vi "Initialize Daemon.vi"(8 "error in":errorcluster, 9 "Data Model":refnum<class "Device Data Model.lvclass">, 10 "transmission data unit":refnum<class "Transmission Data Unit.lvclass">, 11 "TCP slave in":refnum<class "TCP Slave.lvclass">) -> (0 "error out":errorcluster, 3 "TCP slave out":refnum<class "TCP Slave.lvclass">)   [LabVIEW 2012, in "TCP Slave.lvclass"]
doc: "Launches the connection daemon and creates the notifier which will allow it to quit."
uses:
  TCP Slave.lvclass
  Transmission Data Unit/Transmission Data Unit.lvclass
  Data Model/Device Data Model.lvclass
  Connection Counter.ctl
  Connection.ctl
  TCP Slave.lvclass/TCP Slave.ctl
  Network Slave.lvclass
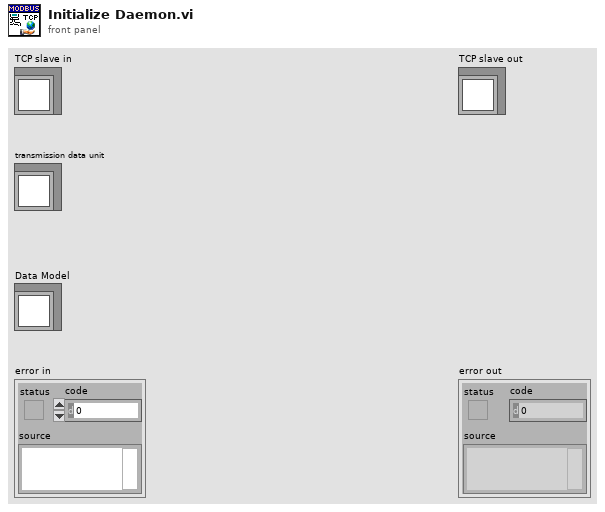
[diagram p1: front panel]
types:
  T1 = typedef "TCP Slave.lvclass/Connection Counter.ctl" = cluster{"Currently Connected":u32, "Connection Records":refnum<data-value>[]}
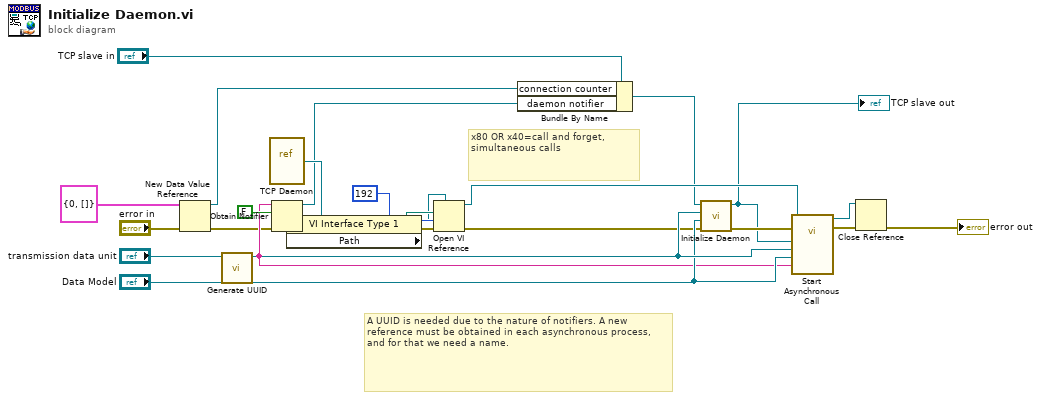
[diagram p0: block diagram]
diagram:
  # "x80 OR x40=call and forget, simultaneous calls"
  # "A UUID is needed due to the nature of notifiers. A new reference must be obtained in each asynchronous process, and for that we need a name."
  n1 = New Data Value Reference(data value=T1 {"Currently Connected"=0, "Connection Records"=[]} ("Connection Counter"), error in="error in") -> (data value reference=w5:refnum<data-value>, error out=w6:errorcluster)
  n2 = call "Generate UUID.vi"() -> ("UUID"=w12:string)  [unwired: 11 in]
  n3 = vi-ref "TCP Daemon.vi"() -> (w20:refnum<vi>)
  n4 = Obtain Notifier(name (unnamed)=w12, notification data type=FALSE, error in (no error)=w6) -> (notifier out=w13:refnum<notifier>, error out=w15:errorcluster)  [unwired: 1 in, 1 out]
  n5 = property class="VI Interface Type 1"(reference=w20, error in=w15) -> (reference out=w1:refnum<vi>, error out=w19:errorcluster, "Path"=w18:path)
  n6 = Open VI Reference(type specifier VI Refnum (for type only)=w1, vi path=w18, options=192 ("x .or. y?"), error in (no error)=w19) -> (vi reference=w17:refnum<vi>, error out=w9:errorcluster)  [unwired: 2 in]
  n7 = Bundle By Name(cluster="TCP slave in", "connection counter"=w5, "daemon notifier"=w13) -> (w10:refnum<class "TCP Slave.lvclass">)
  n8 = call-parent "Initialize Daemon.vi"("error in"=w9, "Data Model"="Data Model", "transmission data unit"="transmission data unit", "network slave in"=w10) -> ("error out"=w11:errorcluster, "network slave out"=w8:refnum<class "TCP Slave.lvclass">)  [unwired: 6 in]
  "TCP slave out" <- w8
  n9 = call-by-ref "Start Asynchronous Call"(reference=w17, error in=w11, "UUID"=w12, "Data Model"="Data Model", "transmission data unit"="transmission data unit", "TCP slave in"=w8) -> (reference out=w2:refnum<vi>, error out=w23:errorcluster)  [unwired: 8 in]
  n10 = Close Reference(reference=w2, error in (no error)=w23) -> (error out=→"error out":errorcluster)
